vi "01 - Acquire Analyze Present.vi"() -> ()   [LabVIEW 2025]
uses:
  <vilib>/express/express analysis/Spectral/Block/exnSpectralBlock spectral measurements power poly.vi
  <vilib>/express/express analysis/Spectral/Block/exnSpectralBlock spectral measurements power DDT.vi
  <vilib>/addons/Time Frequency Analysis/_control.llb/TFA Configure Spectrogram Indicator (Predefined Color Table).vi
  <vilib>/express/express analysis/Spectral/XNode/ExpressSpectralMeasurementsBlockNode.xnode
  <vilib>/addons/_Advanced Signal Processing/NI_AdvSigProcTFA.lvlib
panel:
  in  "Lower Cutoff, Hz":dbl=1600.0 format="%.3p"
  in  "Acquisition Duration, sec":dbl=3.0 format="%#_13g"
  out "Time Domain":dynamicdata(graph)
  out "Power Spectrum":dynamicdata(graph)
  out "Spectrogram":dbl[][](graph)
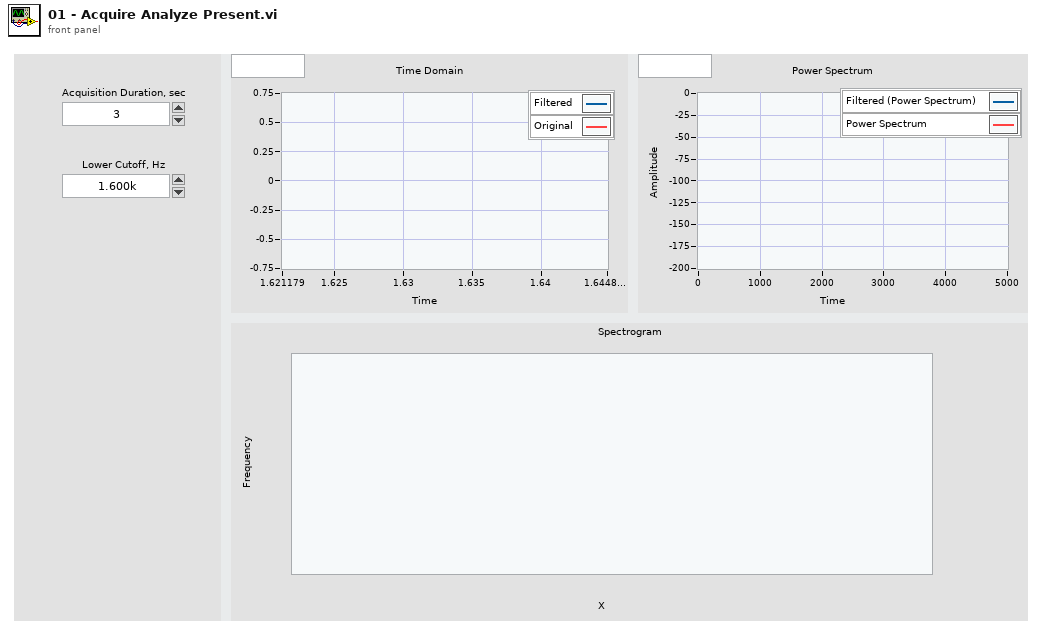
[diagram p1: front panel]
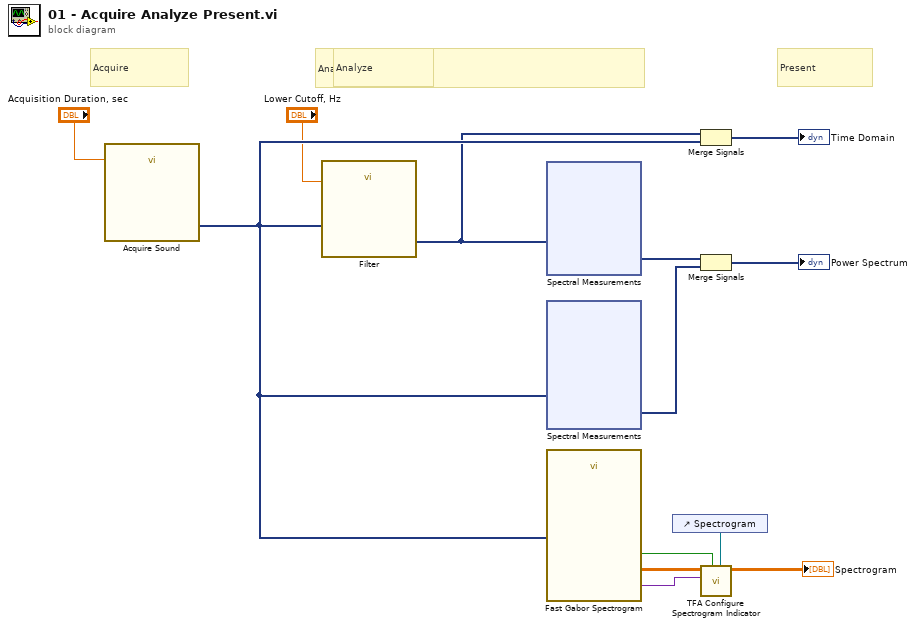
[diagram p0: block diagram]
diagram:
  # "Analyze"
  # "Present"
  # "Analyze"
  # "Acquire"
  n1 = call "Acquire Sound"("Duration (s)"="Acquisition Duration, sec") -> ("Data"=w9:dynamicdata)  [unwired: 17 in, 1 out]
  n2 = call "Filter"("Lower Cut-Off"="Lower Cutoff, Hz", "Signal"=w9) -> ("Filtered Signal"=w4:dynamicdata)  [unwired: 8 in, 1 out]
  n3 = xnode "Spectral Measurements"("Signals"=w4) -> ("Power Spectrum"=w6:dynamicdata)  [unwired: 1 in, 1 out]
  n4 = xnode "Spectral Measurements"("Signals"=w9) -> ("Power Spectrum"=w7:dynamicdata)  [unwired: 1 in, 1 out]
  n5 = call "Fast Gabor Spectrogram"("Signal"=w9) -> ("Scale Info"=w3:variant, "Spectrogram"=w13:dbl[][], "dB"=w10:bool)  [unwired: 6 in, 2 out]
  n6 = control-ref of="Spectrogram"() -> (w11:refnum<vi>)
  n7 = Merge Signals(w4, w9) -> (→"Time Domain":dynamicdata)
  n8 = Merge Signals(w6, w7) -> (→"Power Spectrum":dynamicdata)
  n9 = call-poly <vilib>:"TFA Configure Spectrogram Indicator.vi"("reference of TF spectrogram indicator"=w11, "dB on? (F)"=w10, "scale info"=w3, "spectrogram"=w13) -> ("TF spectrogram indicator"=→"Spectrogram":dbl[][])  [unwired: 6 in, 1 out]
